vi "Gateway_Listen.vi"(8 "error in (no error)":errorcluster, 11 "GatewayClass in":refnum<class "GatewayClass.lvclass">) -> (0 "error out":errorcluster, 2 "Next Step":T1, 3 "GatewayClass out":refnum<class "GatewayClass.lvclass">)   [LabVIEW 2018, in "GatewayClass.lvclass"]
uses:
  GatewayClass.lvclass
  Gateway_States.ctl
  GatewayClass.lvclass/GatewayClass.ctl
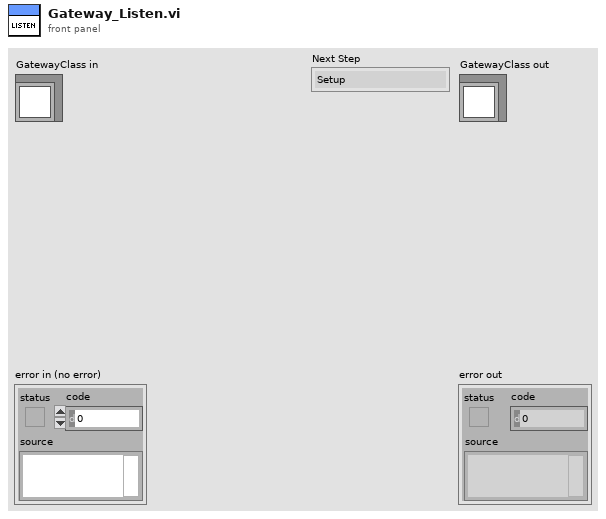
[diagram p1: front panel]
types:
  T1 = typedef "Gateway_States.ctl" = enum16{"Setup", "Connnect", "Initialise", "Close", "Listen", "Send", "RecodeJson", "Reply", ""}
  T2 = enum16{"big-endian, network order", "native, host order", "little-endian"}
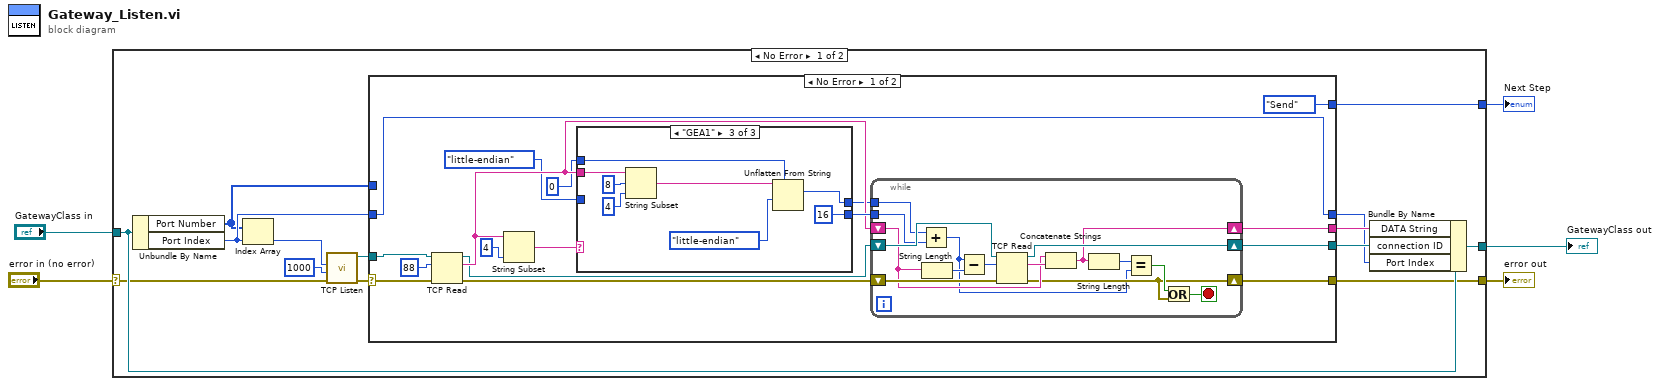
[diagram p0: block diagram]
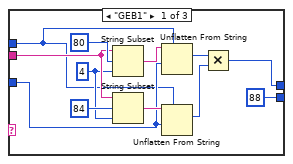
[diagram p2: hidden frame]
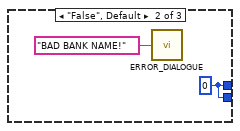
[diagram p3: hidden frame]
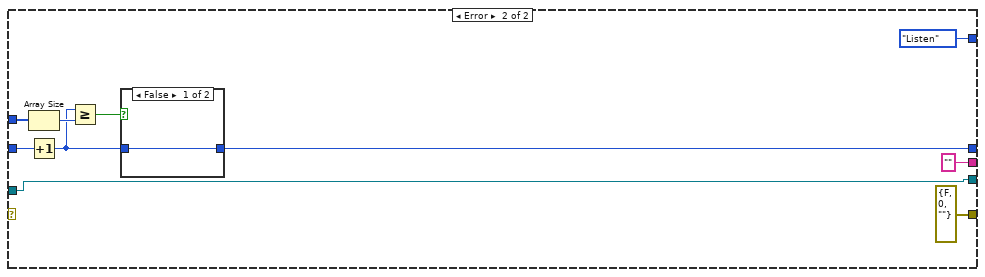
[diagram p4: hidden frame]
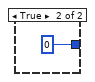
[diagram p5: hidden frame]
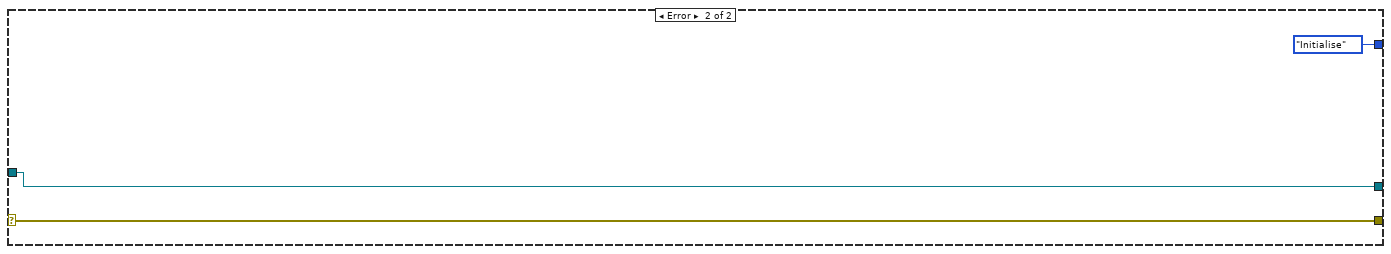
[diagram p6: hidden frame]
diagram:
  n1 = case shown="No Error" "error in (no error)" {
    selector: "error in (no error)" -> [w10 w88]
    tunnel: [w9 w88] -> w4
    tunnel: [w12 w87] -> w2
    tunnel: "GatewayClass in" -> [w14 w87]
    tunnel: [w15 Gateway_States."Initialise"] -> w1
    frame No Error {
      n2 = Unbundle By Name(w14) -> ("Port Number"=w7:u16[], "Port Index"=w8:i32)
      n3 = Index Array(array=w7, index=w8) -> (element=w16:u16)
      n4 = call <vilib>:"TCP Listen.vi"("error in (no error)"=w10, "timeout ms (wait forever: -1)"=1000, "port"=w16) -> ("error out"=w18:errorcluster, "connection ID"=w19:refnum<k5>)  [unwired: 4 in, 3 out]
      n5 = case shown="No Error" w18 {
        selector: w18 -> [w21 _]
        tunnel: [Gateway_States."Send" Gateway_States."Listen"] -> w15
        tunnel: w19 -> [w25 w82]
        tunnel: [w24 errorcluster {"status"=FALSE, "code"=0, "source"=""} ("error out")] -> w9
        tunnel: [w23 "" ("data out")] -> w13
        tunnel: [w22 w82] -> w11
        tunnel: w8 -> [w20 w76]
        tunnel: w7 -> [_ w75]
        tunnel: [w20 w74] -> w6
        frame No Error {
          n6 = TCP Read(connection ID=w25, bytes to read=88, error in (no error)=w21) -> (connection ID out=w29:refnum<k5>, data out=w34:string, error out=w33:errorcluster)  [unwired: 2 in]
          n7 = String Subset(string=w34, length (rest)=4 ("length (rest)")) -> (substring=w28:string)  [unwired: 1 in]
          n8 = case shown="\"GEA1\"" w28 {
            tunnel: w34 -> [w61 _ w71]
            tunnel: u32 0 -> [w56 _ w70]
            tunnel: T2."little-endian" ("byte order (0:big-endian, network order)") -> [w57 _ _]
            tunnel: [w53 w64 w67] -> w32
            tunnel: [u32 88 ("y") w64 u32 16 ("y")] -> w35
            frame "GEB1" {
              w59 = 4 ("length (rest)")
              n9 = String Subset(string=w61, offset (0)=80, length (rest)=w59) -> (substring=w62:string)
              n10 = String Subset(string=w61, offset (0)=84, length (rest)=w59) -> (substring=w58:string)
              n11 = Unflatten From String(type=w56, binary string=w62, byte order (0:big-endian, network order)=w57) -> (value=w54:u32)  [unwired: 2 in, 2 out]
              n12 = Unflatten From String(type=w56, binary string=w58, byte order (0:big-endian, network order)=w57) -> (value=w55:u32)  [unwired: 2 in, 2 out]
              n13 = Multiply(x=w54, y=w55) -> (x*y=w53:u32)
            }
            frame "False", Default {
              w64 = u32 0
              n14 = call "ERROR_DIALOGUE.vi"("String"="BAD BANK NAME!") -> ()
            }
            frame "GEA1" {
              n15 = String Subset(string=w71, offset (0)=8, length (rest)=4 ("length (rest)")) -> (substring=w69:string)
              n16 = Unflatten From String(type=w70, binary string=w69, byte order (0:big-endian, network order)=T2."little-endian") -> (value=w67:u32)  [unwired: 2 in, 2 out]
            }
          }
          n17 = while {
            tunnel: w32 -> [w39]
            shift-right: [w49] -> w22
            shift-left: w29 -> [w51]
            shift-right: [w45] -> w23
            shift-left: w34 -> [w47]
            shift-right: [w42] -> w24
            shift-left: w33 -> [w48]
            tunnel: w35 -> [w37]
            stop <- w41 stop-if-true
            n18 = Add(x=w39, y=w37) -> (x+y=w38:u32)
            n19 = String Length(string=w47) -> (length=w40:i32)
            n20 = Subtract(x=w38, y=w40) -> (x-y=w46:u32)
            n21 = TCP Read(connection ID=w51, bytes to read=w46, error in (no error)=w48) -> (connection ID out=w49:refnum<k5>, data out=w50:string, error out=w42:errorcluster)  [unwired: 2 in]
            n22 = Concatenate Strings(w47, w50) -> (w45:string)
            n23 = String Length(string=w45) -> (length=w44:i32)
            n24 = Equal?(x=w44, y=w38) -> (x = y?=w43:bool)
            n25 = Or(x=w43, y=w42) -> (x .or. y?=w41:bool)
          }
        }
        frame Error {
          n26 = Array Size(array=w75) -> (size(s)=w78:i32)
          n27 = Increment(x=w76) -> (x+1=w77:i32)
          n28 = Greater Or Equal?(x=w77, y=w78) -> (x >= y?=w79:bool)
          n29 = case shown="False" w79 {
            tunnel: [w84 0] -> w74
            tunnel: w77 -> [w84 _]
            frame False {
            }
            frame True {
            }
          }
        }
      }
      n30 = Bundle By Name(cluster=w14, "DATA String"=w13, "connection ID"=w11, "Port Index"=w6) -> (w12:refnum<class "GatewayClass.lvclass">)
    }
    frame Error {
    }
  }
  "error out" <- w4
  "GatewayClass out" <- w2
  "Next Step" <- w1
